vi "One Detected.vi"(8 "error in (no error)":errorcluster, 10 "Targets in":T7 {"Filtered Targets"."IP Mode" items=["Static"=1, "DHCP/Link-Local"=2, "Link-Local Only"=4, "DHCP Only"=8]}, 11 "Ctl Refs in":T1) -> (0 "error out":errorcluster, 2 "Targets out":T7 {"Filtered Targets"."IP Mode" items=["Static"=1, "DHCP/Link-Local"=2, "Link-Local Only"=4, "DHCP Only"=8]}, 3 "Ctl Refs out":T1)   [LabVIEW 2013]
uses:
  Controls/Refs.ctl
  Controls/Button Refs.ctl
  Controls/Tab Ctl Refs.ctl
  types/TabStateType.ctl
  Controls/Indicator Refs.ctl
  Controls/Slider Refs.ctl
  Controls/Control Refs.ctl
  Controls/Targets.ctl
  Controls/Detected.ctl
  types/MAX Sys Cfg Target Information.ctl
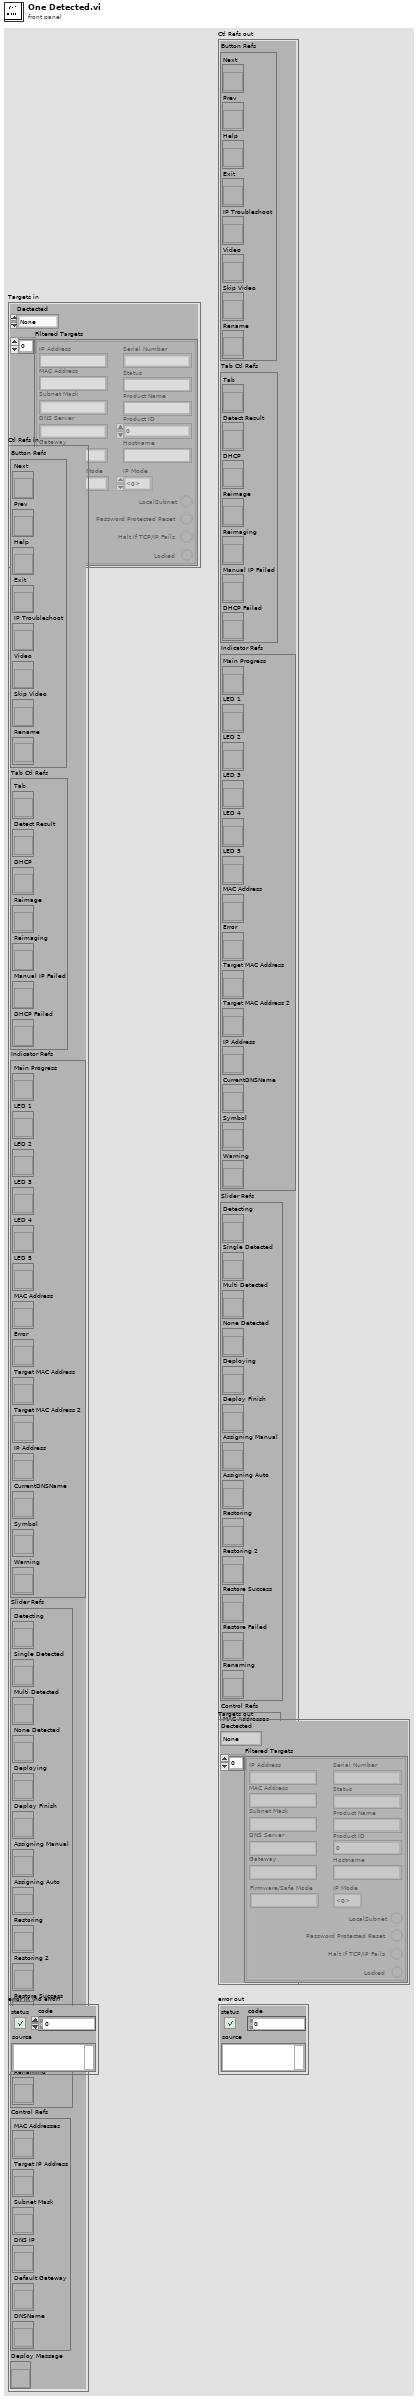
[diagram p1: front panel]
types:
  T1 = typedef "Refs.ctl" = cluster{"Button Refs":T2, "Tab Ctl Refs":T3, "Indicator Refs":T4, "Slider Refs":T5, "Control Refs":T6, "Deploy Message":refnum<vi>}
  T2 = typedef "Button Refs.ctl" = cluster{"Next":refnum<vi>, "Prev":refnum<vi>, "Help":refnum<vi>, "Exit":refnum<vi>, "IP Troubleshoot":refnum<vi>, "Video":refnum<vi>, "Skip Video":refnum<vi>, "Rename":refnum<vi>}
  T3 = typedef "Tab Ctl Refs.ctl" = cluster{"Tab":refnum<vi>, "Detect Result":refnum<vi>, "DHCP":refnum<vi>, "Reimage":refnum<vi>, "Reimaging":refnum<vi>, "Manual IP Failed":refnum<vi>, "DHCP Failed":refnum<vi>}
  T4 = typedef "Indicator Refs.ctl" = cluster{"Main Progress":refnum<vi>, "LED 1":refnum<vi>, "LED 2":refnum<vi>, "LED 3":refnum<vi>, "LED 4":refnum<vi>, "LED 5":refnum<vi>, "MAC Address":refnum<vi>, "Error":refnum<vi>, "Target MAC Address":refnum<vi>, "Target MAC Address 2":refnum<vi>, "IP Address":refnum<vi>, "CurrentDNSName":refnum<vi>, "Symbol":refnum<vi>, "Warning":refnum<vi>}
  T5 = typedef "Slider Refs.ctl" = cluster{"Detecting":refnum<vi>, "Single Detected":refnum<vi>, "Multi Detected":refnum<vi>, "None Detected":refnum<vi>, "Deploying":refnum<vi>, "Deploy Finish":refnum<vi>, "Assigning Manual":refnum<vi>, "Assigning Auto":refnum<vi>, "Restoring":refnum<vi>, "Restoring 2":refnum<vi>, "Restore Success":refnum<vi>, "Restore Failed":refnum<vi>, "Renaming":refnum<vi>}
  T6 = typedef "Control Refs.ctl" = cluster{"MAC Addresses":refnum<vi>, "Target IP Address":refnum<vi>, "Subnet Mask":refnum<vi>, "DNS IP":refnum<vi>, "Default Gateway":refnum<vi>, "DNSName":refnum<vi>}
  T7 = typedef "Targets.ctl" = cluster{"Dectected":T8, "Filtered Targets":T9[]}
  T8 = typedef "Detected.ctl" = enum16{"None", "Failed", "Single", "Multi"}
  T9 = typedef "MAX Sys Cfg Target Information.ctl" = cluster{"MAC Address":string, "IP Address":string, "Status":string, "Product Name":string, "Hostname":string, "Firmware/Safe Mode":string, "Subnet Mask":string, "Gateway":string, "DNS Server":string, "Serial Number":string, "Product ID":u32, "Locked ":bool, "LocalSubnet":bool, "Halt If TCP/IP Fails":bool, "Password Protected Reset":bool, "IP Mode":i32}
  T10 = typedef "TabStateType.ctl" = enum32{"Welcome", "Instructions", "Detect", "Run Detection", "Detect Result", "Deploy", "Run Deployment", "Connect Verify", "Success", "DHCP", "Troubleshoot", "System Restore", "Error", "Video", "Rename"}
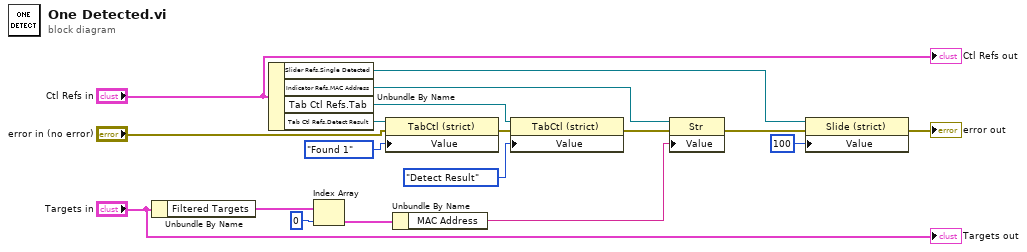
[diagram p0: block diagram]
diagram:
  n1 = Unbundle By Name("Targets in") -> ("Filtered Targets"=w6:T9[])
  n2 = Unbundle By Name("Ctl Refs in") -> ("Slider Refs.Single Detected"=w3:refnum<vi>, "Indicator Refs.MAC Address"=w4:refnum<vi>, "Tab Ctl Refs.Tab"=w7:refnum<vi>, "Tab Ctl Refs.Detect Result"=w8:refnum<vi>)
  n3 = Index Array(array=w6, index=0) -> (element=w10:T9)
  n4 = property on="Property Node" class="TabCtl (strict)"(reference=w8, error in="error in (no error)", "Value"=enum32{"Found 0", "Found 1", "Found 2"}."Found 1" ("Detect Result Tabs")) -> (error out=w14:errorcluster)  [unwired: 1 out]
  n5 = Unbundle By Name(w10) -> ("MAC Address"=w9:string)
  n6 = property on="Property Node" class="TabCtl (strict)"(reference=w7, error in=w14, "Value"=TabStateType."Detect Result" ("Tab Control")) -> (error out=w5:errorcluster)  [unwired: 1 out]
  n7 = property on="Property Node" class="Str"(reference=w4, error in=w5, "Value"=w9) -> (error out=w2:errorcluster)  [unwired: 1 out]
  n8 = property on="Property Node" class="Slide (strict)"(reference=w3, error in=w2, "Value"=i8 100 ("Slide 4")) -> (error out=→"error out":errorcluster)  [unwired: 1 out]
  "Ctl Refs out" <- "Ctl Refs in"
  "Targets out" <- "Targets in"
